vi "Proyecto_Final_v3.vi"() -> ()   [LabVIEW 2021]
uses:
  <vilib>/Instr/_visa.llb/VISA Configure Serial Port (Instr).vi
panel:
  out "read buffer":string
  in  "baud rate (9600)":u32=9600
  in  "Puerto Serial":refnum<visa-resource-name>
  in  "Boolean":bool
  in  "Ingresar":bool
  in  "Password":string
  in  "Username":string
  out "Acceso":bool
  out "Ventana":bool
  in  "Temperatura":dbl
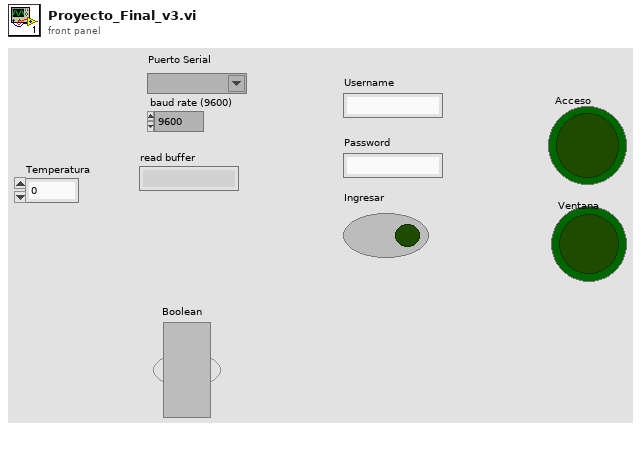
[diagram p1: front panel]
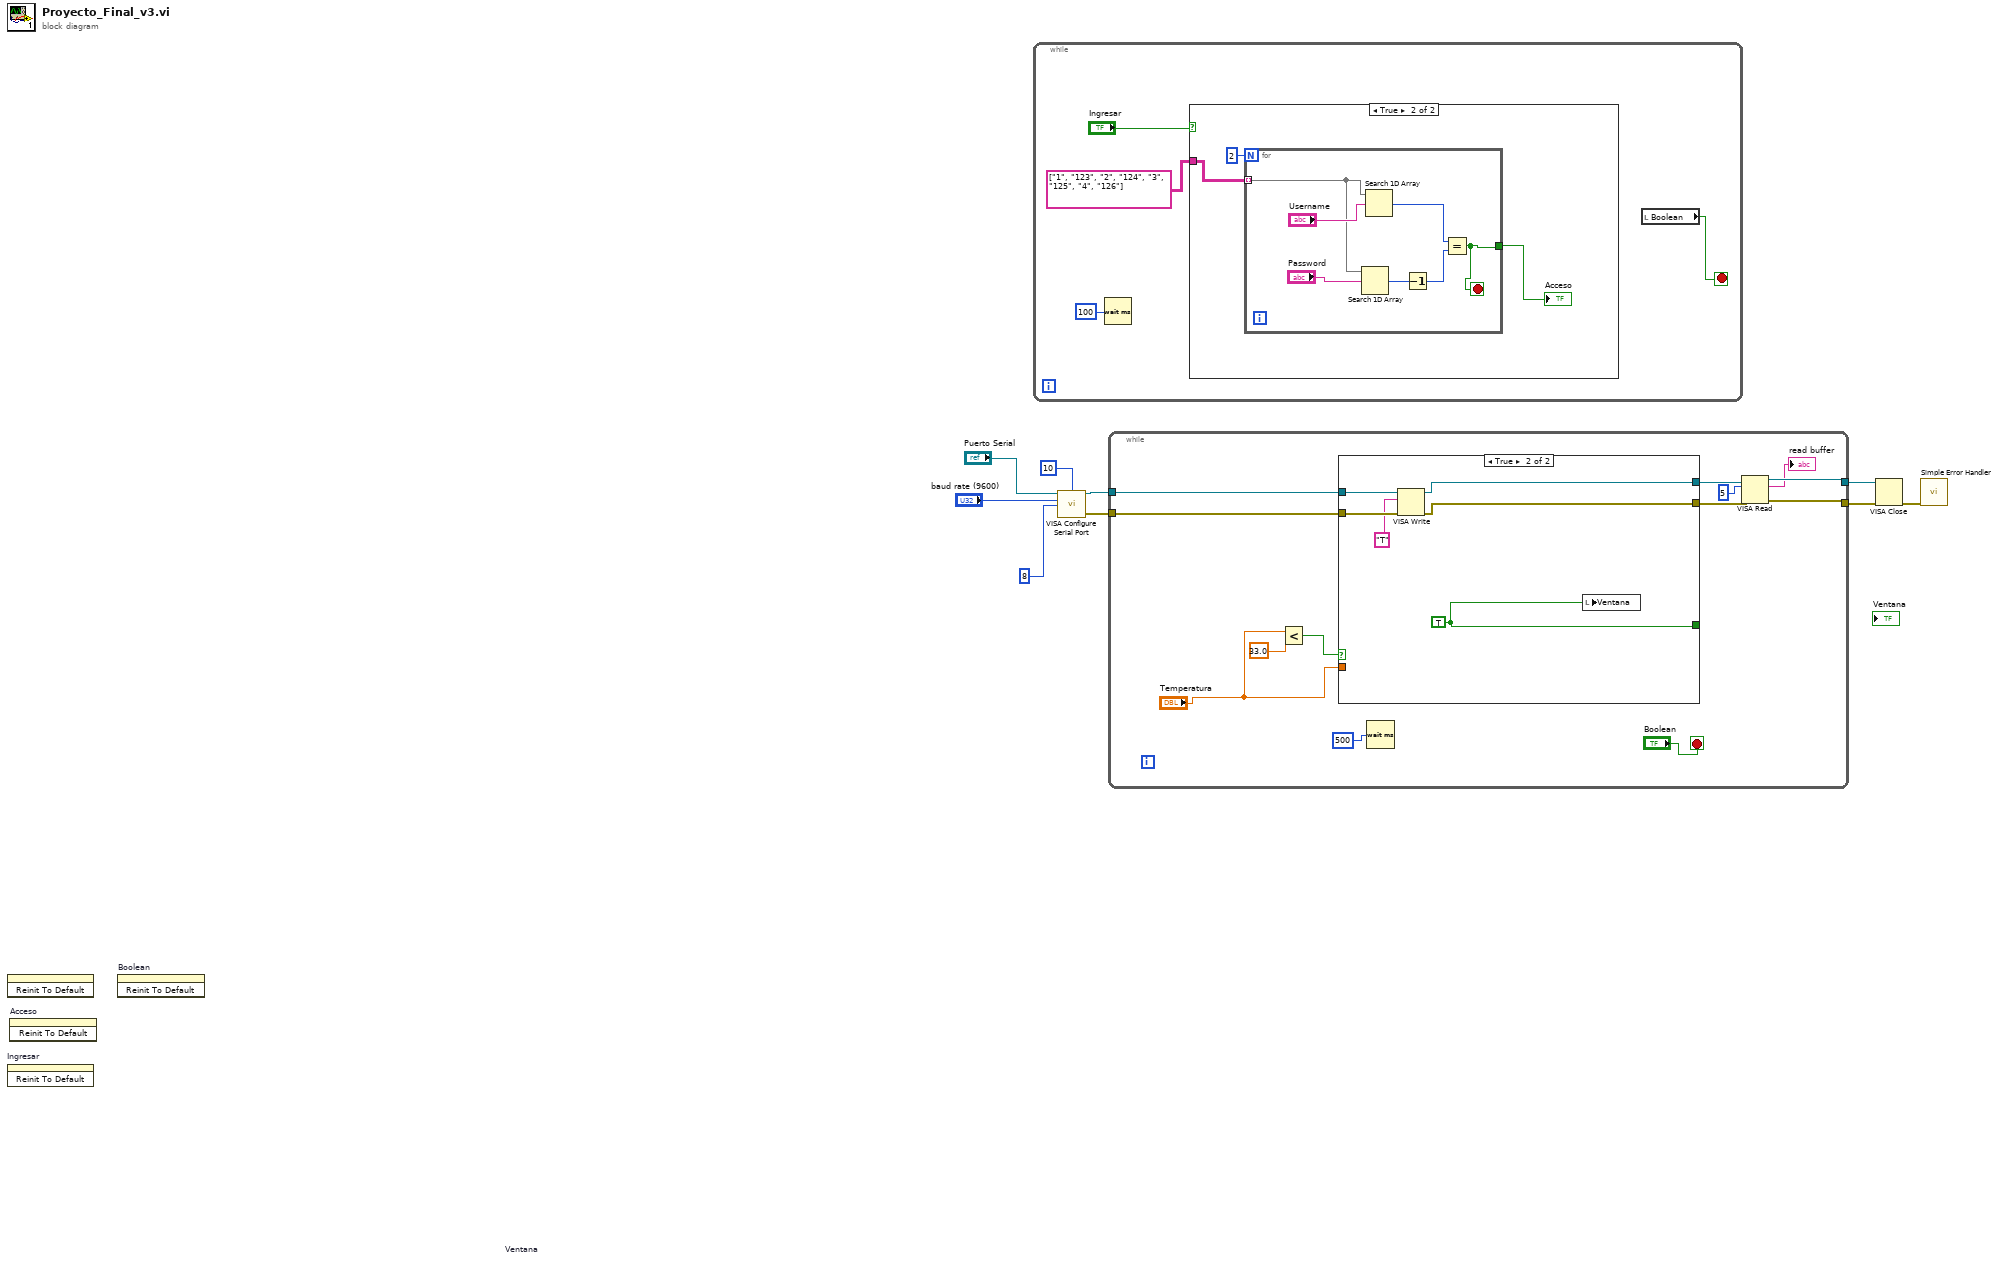
[diagram p0: block diagram]
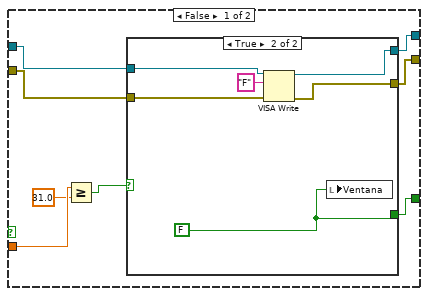
[diagram p3: hidden frame]
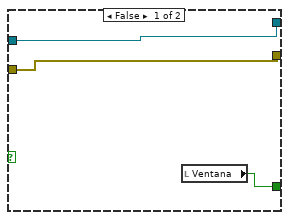
[diagram p4: hidden frame]
diagram:
  n1 = invoke on="Ventana" class="Bool (strict)" method="Reinit To Default"() -> ()  [unwired: 3 in, 3 out]
  n2 = invoke on="Ingresar" class="Bool (strict)" method="Reinit To Default"() -> ()  [unwired: 3 in, 3 out]
  n3 = invoke on="Acceso" class="Bool (strict)" method="Reinit To Default"() -> ()  [unwired: 3 in, 3 out]
  n4 = invoke on="Boolean" class="Bool (strict)" method="Reinit To Default"() -> ()  [unwired: 3 in, 3 out]
  n5 = while {
    stop <- w10 stop-if-true
    n6 = Wait (ms)(milliseconds to wait=u32 100) -> ()  [unwired: 1 out]
    n7 = case shown="True" "Ingresar" {
      tunnel: string[][] [["1", "123"], ["2", "124"], ["3", "125"], ["4", "126"]] ("array") -> [_ w15]
      frame False {
      }
      frame True {
        n8 = for {
          N: 2 -> [_]
          tunnel: w15 -> [w21] mode=indexing
          tunnel: [w17] -> w14
          stop <- w17 stop-if-true
          n9 = Search 1D Array(1D array=w21, element="Password") -> (index of element=w19:i32)  [unwired: 1 in]
          n10 = Search 1D Array(1D array=w21, element="Username") -> (index of element=w20:i32)  [unwired: 1 in]
          n11 = Decrement(x=w19) -> (x-1=w18:i32)
          n12 = Equal?(x=w20, y=w18) -> (x = y?=w17:bool)
        }
        "Acceso" <- w14
      }
    }
    n13 = local read "Boolean"() -> (w10:bool)
  }
  n14 = call-poly "VISA Configure Serial Port"("VISA resource name"="Puerto Serial", "termination char\n(0xA = '\\n' = LF)"=u8 10 ("termination char\n(0xA = '\\n' = LF)"), "baud rate (9600)"="baud rate (9600)", "data bits (8)"=u16 8) -> ("VISA resource name out"=w4:refnum<visa-resource-name>, "error out"=w3:errorcluster)  [unwired: 10 in]
  n15 = while {
    tunnel: w4 -> [w31]
    tunnel: w3 -> [w30]
    tunnel: [w27] -> w2
    tunnel: [w26] -> w1
    stop <- "Boolean" stop-if-true
    n16 = Less?(x="Temperatura", y=33.0) -> (x < y?=w34:bool)
    n17 = case shown="True" w34 {
      tunnel: "Temperatura" -> [w44 _]
      tunnel: [w42 w59] -> _
      tunnel: w31 -> [w40 w58]
      tunnel: w30 -> [w39 w57]
      tunnel: [w38 w56] -> w29
      tunnel: [w37 w55] -> w28
      frame False {
        n18 = Greater Or Equal?(x=w44, y=31.0) -> (x >= y?=w41:bool)
        n19 = case shown="True" w41 {
          tunnel: [w47 w53] -> w42
          tunnel: w40 -> [w46 w51]
          tunnel: w39 -> [w45 w50]
          tunnel: [w46 w48] -> w38
          tunnel: [w45 w49] -> w37
          frame False {
            n20 = local read "Ventana"() -> (w47:bool)
          }
          frame True {
            w53 = FALSE
            n21 = VISA Write(VISA resource name=w51, write buffer="F", error in (no error)=w50) -> (VISA resource name out=w48:refnum<visa-resource-name>, error out=w49:errorcluster)  [unwired: 1 out]
            n22 = local write "Ventana"(w53) -> ()
          }
        }
      }
      frame True {
        w59 = TRUE
        n23 = VISA Write(VISA resource name=w58, write buffer="T", error in (no error)=w57) -> (VISA resource name out=w56:refnum<visa-resource-name>, error out=w55:errorcluster)  [unwired: 1 out]
        n24 = local write "Ventana"(w59) -> ()
      }
    }
    n25 = Wait (ms)(milliseconds to wait=u32 500) -> ()  [unwired: 1 out]
    n26 = VISA Read(VISA resource name=w29, byte count=u32 5, error in (no error)=w28) -> (VISA resource name out=w27:refnum<visa-resource-name>, read buffer=→"read buffer":string, error out=w26:errorcluster)  [unwired: 1 out]
  }
  n27 = VISA Close(VISA resource name=w2, error in (no error)=w1) -> (error out=w5:errorcluster)
  n28 = call <vilib>:"Simple Error Handler.vi"("error in (no error)"=w5) -> ()  [unwired: 4 in, 5 out]
